vi "GetPortSelection.vi"(6 "Port":i32, 9 "ConnTypes":string[](array[string])=["A", "B", "C"]) -> (1 "Combo Box 2":string="Make Selection")   [LabVIEW 2018, in "PNA-X.lvlib"]
uses:
  PNA-X.lvlib
panel:
  out "Present Port":i32
  in  "Connector Type Selection":string(combo)="Make Selection"
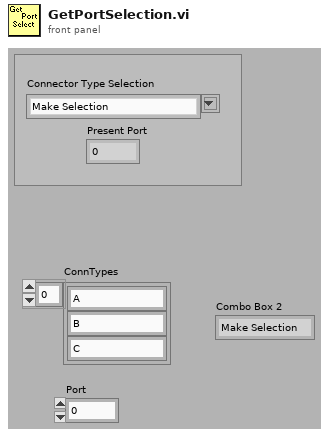
[diagram p1: front panel]
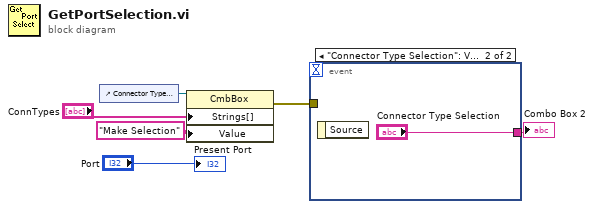
[diagram p0: block diagram]
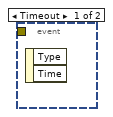
[diagram p2: hidden frame]
diagram:
  n1 = control-ref of="Connector Type Selection"() -> (w6:refnum<vi>)
  n2 = property class="CmbBox"(reference=w6, "Strings[]"="ConnTypes", "Value"="Make Selection") -> (error out=w5:errorcluster)  [unwired: 1 in, 1 out]
  n3 = event shown="[1] \"Connector Type Selection\": Value Change" {
    selector: _ -> [_ _]
    dyn-events: _ -> [_ _]
    timeout: _ -> [_ _]
    tunnel: w5 -> [_ _]
    tunnel: [_ "Connector Type Selection"] -> w4
    event Timeout {
      n4 = event-data() -> ()  [unwired: 1 in, 2 out]
    }
    event "Connector Type Selection": Value Change {
      n5 = event-data() -> ()  [unwired: 1 in, 1 out]
    }
  }
  "Combo Box 2" <- w4
  "Present Port" <- "Port"
